vi "Read Y_state.vi"(8 "error in (no error)":errorcluster, 11 "Y_H in":refnum<class "Y_H.lvclass">) -> (0 "error out":errorcluster, 2 "button state":T1, 3 "Y_H out":refnum<class "Y_H.lvclass">)   [LabVIEW 2019, in "Y_H.lvclass"]
uses:
  Y_H.lvclass
  ctl/Y_H_state.ctl
  Y_H.lvclass/Y_H.ctl
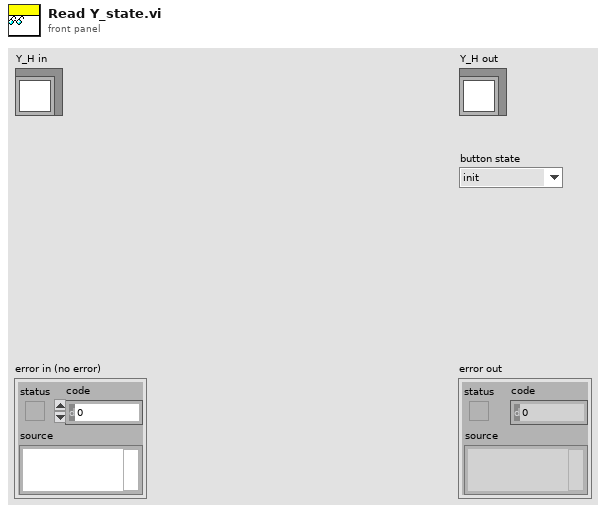
[diagram p1: front panel]
types:
  T1 = typedef "Y_H.lvclass/Y_H_state.ctl" = enum16{"init", "value change", "value not changed"}
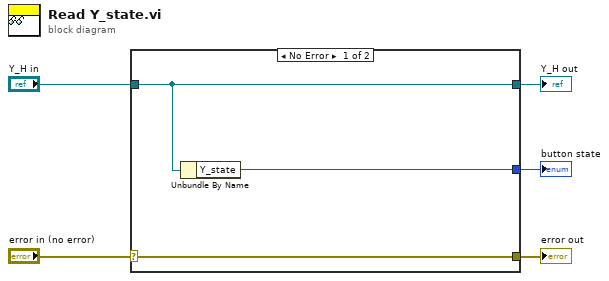
[diagram p0: block diagram]
diagram:
  n1 = case shown="No Error" "error in (no error)" {
    selector: "error in (no error)" -> [w8 w9]
    tunnel: [w8 w9] -> w4
    tunnel: [w7 w10] -> w2
    tunnel: "Y_H in" -> [w7 w10]
    tunnel: [w6 _] -> w1
    frame No Error {
      n2 = Unbundle By Name(w7) -> ("Y_state"=w6:T1)
    }
    frame Error {
    }
  }
  "error out" <- w4
  "Y_H out" <- w2
  "button state" <- w1
